vi "serial read parsing mode.vi"() -> ()   [LabVIEW 2020]
uses:
  <vilib>/Instr/_visa.llb/VISA Configure Serial Port (Instr).vi
  <vilib>/Utility/file.llb/Write Delimited Spreadsheet (string).vi
panel:
  out "Cek Parsing":errorcluster
  out "Grafik Suhu Objek":dbl(graph)
  out "Suhu Objek":dbl
  out "Output Suhu Objek":string
  in  "Simpan ke Excel":bool
  out "Grafik BPM ECG":dbl(graph)
  out "Grafik Sinyal Jantung":dbl(graph)
  out "Cek Data Mentah":errorcluster
  in  "Lokasi Penyimpanan Data":path
  out "Output BPM ECG":string
  out "Output Sinyal Jantung":string
  out "Nilai BPM ECG":dbl
  out "Nilai ECG":dbl
  in  "Write Data Serial":string
  in  "Kirim Data":bool
  out "Read Data Serial":string
  in  "STOP":bool
  out "Cek Koneksi":errorcluster
  in  "baud rate (9600)":u32=9600
  in  "PORT kontroler":refnum<visa-resource-name>
  # "MONITORING PENGUKURAN DETAK JANTUNG DAN SUHU TUBUH"
  # "RECEIVER DATA SERIAL"
  # "PARSING DATA SERIAL"
  # "TUGAS AKHIR\n---------------------------------------\nANDRE OKVIRONI\n1711011003\n---------------------------------------\nTEKNIK ELEKTRONIKA INDUSTRI\nPOLITEKNIK NEGERI PADANG"
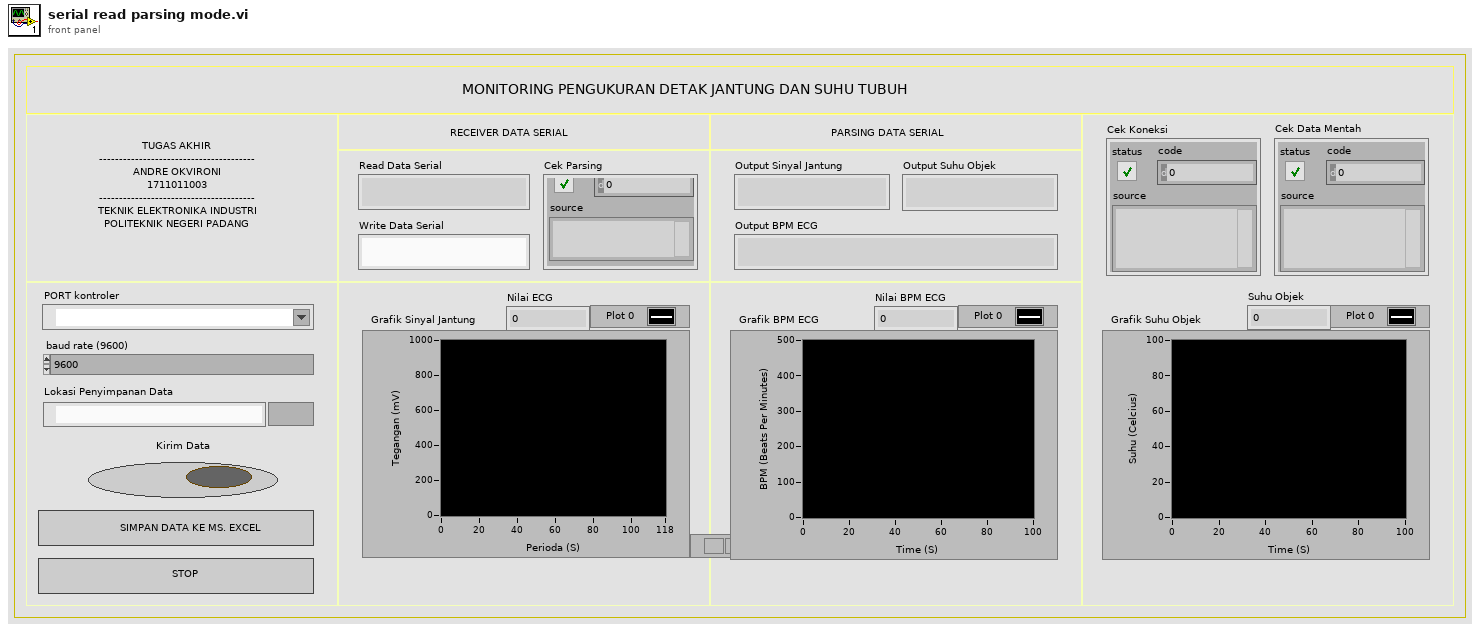
[diagram p1: front panel]
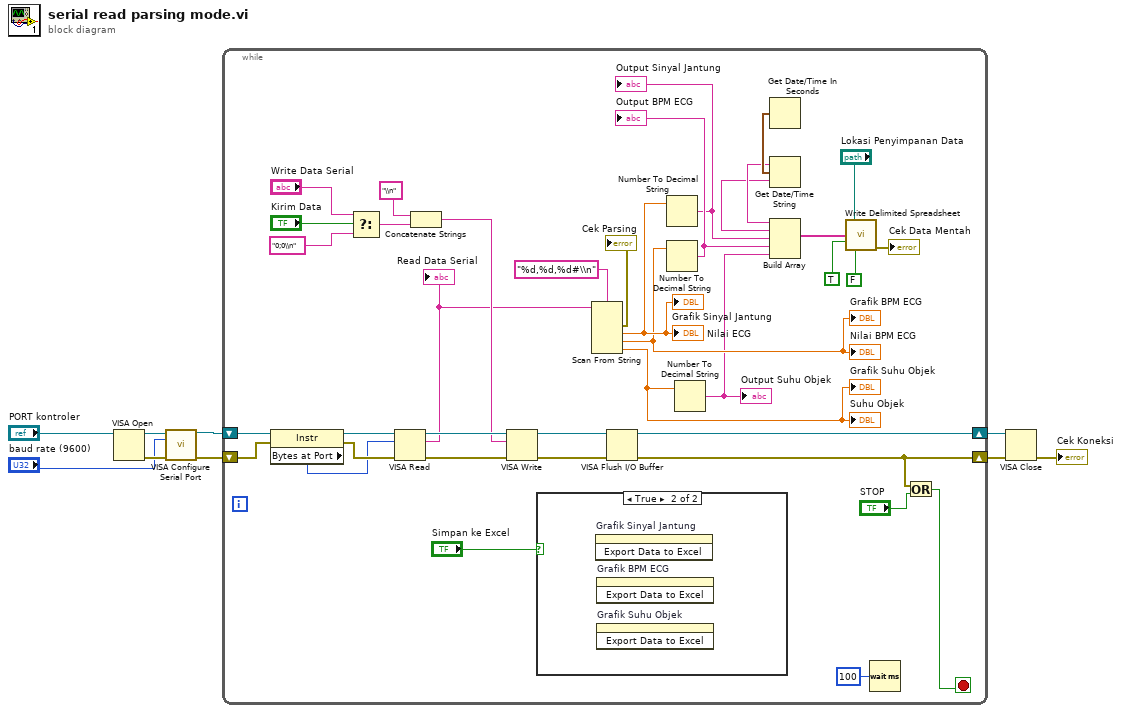
[diagram p0: block diagram]
diagram:
  n1 = VISA Open(VISA resource name="PORT kontroler") -> (VISA resource name=w8:refnum<visa-resource-name>, error out=w7:errorcluster)  [unwired: 4 in]
  n2 = call-poly "VISA Configure Serial Port"("VISA resource name"=w8, "baud rate (9600)"="baud rate (9600)", "error in (no error)"=w7) -> ("VISA resource name out"=w5:refnum<visa-resource-name>, "error out"=w4:errorcluster)  [unwired: 11 in]
  n3 = while {
    shift-right: [w38] -> w3
    shift-left: w5 -> [w47]
    shift-right: [w37] -> w1
    shift-left: w4 -> [w46]
    stop <- w36 stop-if-true
    n4 = property class="Instr"(reference=w47, error in=w46) -> (reference out=w45:refnum<visa-resource-name>, error out=w44:errorcluster, "Bytes at Port"=w43:u32)
    n5 = Select(t="Write Data Serial", s="Kirim Data", f="0;0\\n") -> (s? t:f=w30:string)
    n6 = VISA Read(VISA resource name=w45, byte count=w43, error in (no error)=w44) -> (VISA resource name out=w42:refnum<visa-resource-name>, read buffer=w24:string, error out=w41:errorcluster)  [unwired: 1 out]
    "Read Data Serial" <- w24
    n7 = Concatenate Strings("\\n" ("string"), w30) -> (w28:string)
    n8 = VISA Write(VISA resource name=w42, write buffer=w28, error in (no error)=w41) -> (VISA resource name out=w40:refnum<visa-resource-name>, error out=w39:errorcluster)  [unwired: 1 out]
    n9 = case shown="True" "Simpan ke Excel" {
      frame False {
      }
      frame True {
        n10 = invoke on="Grafik Sinyal Jantung" class="WFChart (strict)" method="Export Data to Excel"() -> ()  [unwired: 3 in, 3 out]
        n11 = invoke on="Grafik BPM ECG" class="WFChart (strict)" method="Export Data to Excel"() -> ()  [unwired: 3 in, 3 out]
        n12 = invoke on="Grafik Suhu Objek" class="WFChart (strict)" method="Export Data to Excel"() -> ()  [unwired: 3 in, 3 out]
      }
    }
    n13 = Scan From String(format string="%d,%d,%d#\\n", input string=w24) -> (error out=→"Cek Parsing":errorcluster, output 1=w16:dbl, output 2=w15:dbl, output 3=w12:dbl)  [unwired: 5 in, 2 out]
    "Nilai ECG" <- w16
    "Nilai BPM ECG" <- w15
    "Grafik Sinyal Jantung" <- w16
    "Grafik BPM ECG" <- w15
    "Suhu Objek" <- w12
    "Grafik Suhu Objek" <- w12
    n14 = VISA Flush I/O Buffer(VISA resource name=w40, error in (no error)=w39) -> (VISA resource name out=w38:refnum<visa-resource-name>, error out=w37:errorcluster)  [unwired: 1 in]
    n15 = Number To Decimal String(number=w16) -> (decimal integer string=w26:string)  [unwired: 1 in]
    "Output Sinyal Jantung" <- w26
    n16 = Number To Decimal String(number=w15) -> (decimal integer string=w27:string)  [unwired: 1 in]
    "Output BPM ECG" <- w27
    n17 = Number To Decimal String(number=w12) -> (decimal integer string=w11:string)  [unwired: 1 in]
    "Output Suhu Objek" <- w11
    n18 = Get Date/Time In Seconds() -> (seconds since 1Jan1904=w25:timestamp)
    n19 = Get Date/Time String(seconds (now)=w25) -> (date string=w23:string, time string=w22:string)  [unwired: 2 in]
    n20 = Build Array(w23, w22, w26, w27, w11) -> (w21:string[])
    n21 = call-poly <vilib>:"Write Delimited Spreadsheet.vi"("file path (dialog if empty)"="Lokasi Penyimpanan Data", "1D data"=w21, "append to file? (new file:F)"=TRUE, "transpose? (no:F)"=FALSE) -> ("error out"=→"Cek Data Mentah":errorcluster)  [unwired: 10 in, 1 out]
    n22 = Wait (ms)(milliseconds to wait=u32 100) -> ()  [unwired: 1 out]
    n23 = Or(x=w37, y="STOP") -> (x .or. y?=w36:bool)
  }
  n24 = VISA Close(VISA resource name=w3, error in (no error)=w1) -> (error out=→"Cek Koneksi":errorcluster)
